vi "发送报文存储-功能全局.vi"(1 "报文输入":string, 10 "枚举":enum16{"ini", "读", "写"}(ring)) -> (15 "报文输出":string)   [LabVIEW 2019]
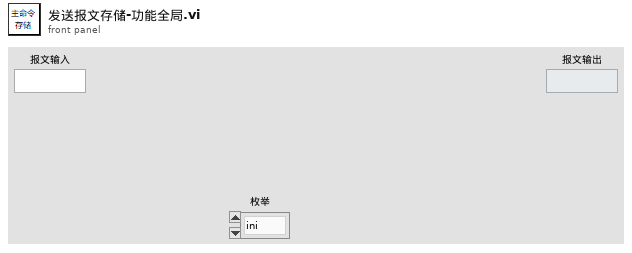
[diagram p1: front panel]
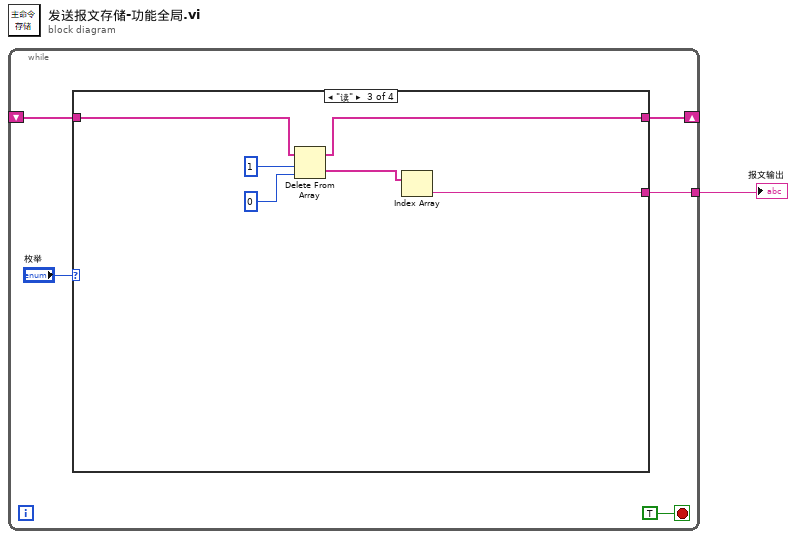
[diagram p0: block diagram]
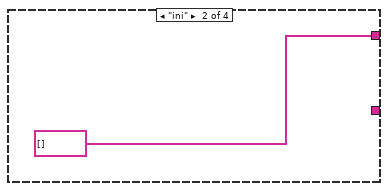
[diagram p3: hidden frame]
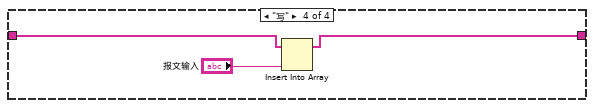
[diagram p4: hidden frame]
diagram:
  n1 = while {
    shift-right: [w4] -> _
    shift-left: _ -> [w3]
    tunnel: [w2] -> w1
    stop <- TRUE stop-if-true
    n2 = case shown="\"读\"" "枚举" {
      tunnel: [w7 string[] [] w13 w16] -> w4
      tunnel: w3 -> [w7 _ w14 w17]
      tunnel: [_ _ w9 _] -> w2
      frame Default {
      }
      frame "ini" {
      }
      frame "读" {
        n3 = Delete From Array(array=w14, length=1 ("长度"), index=0 ("索引")) -> (deleted portion=w10:string[], array with subset deleted=w13:string[])
        n4 = Index Array(array=w10) -> (element=w9:string)  [unwired: 1 in]
      }
      frame "写" {
        n5 = Insert Into Array(array=w17, new element="报文输入") -> (w16:string[])  [unwired: 1 in]
      }
    }
  }
  "报文输出" <- w1
